vi "XNET Fill In Error Info Ex.vi"(0 "error xnet":errorcluster, 11 "error in":errorcluster) -> (15 "error out":errorcluster)   [LabVIEW 2018]
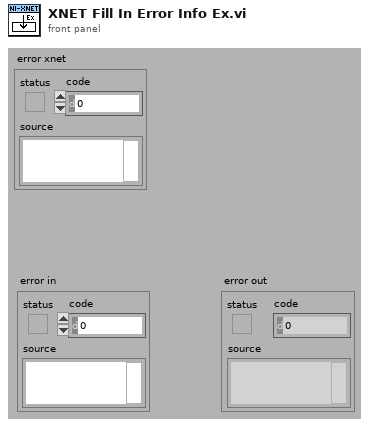
[diagram p1: front panel]
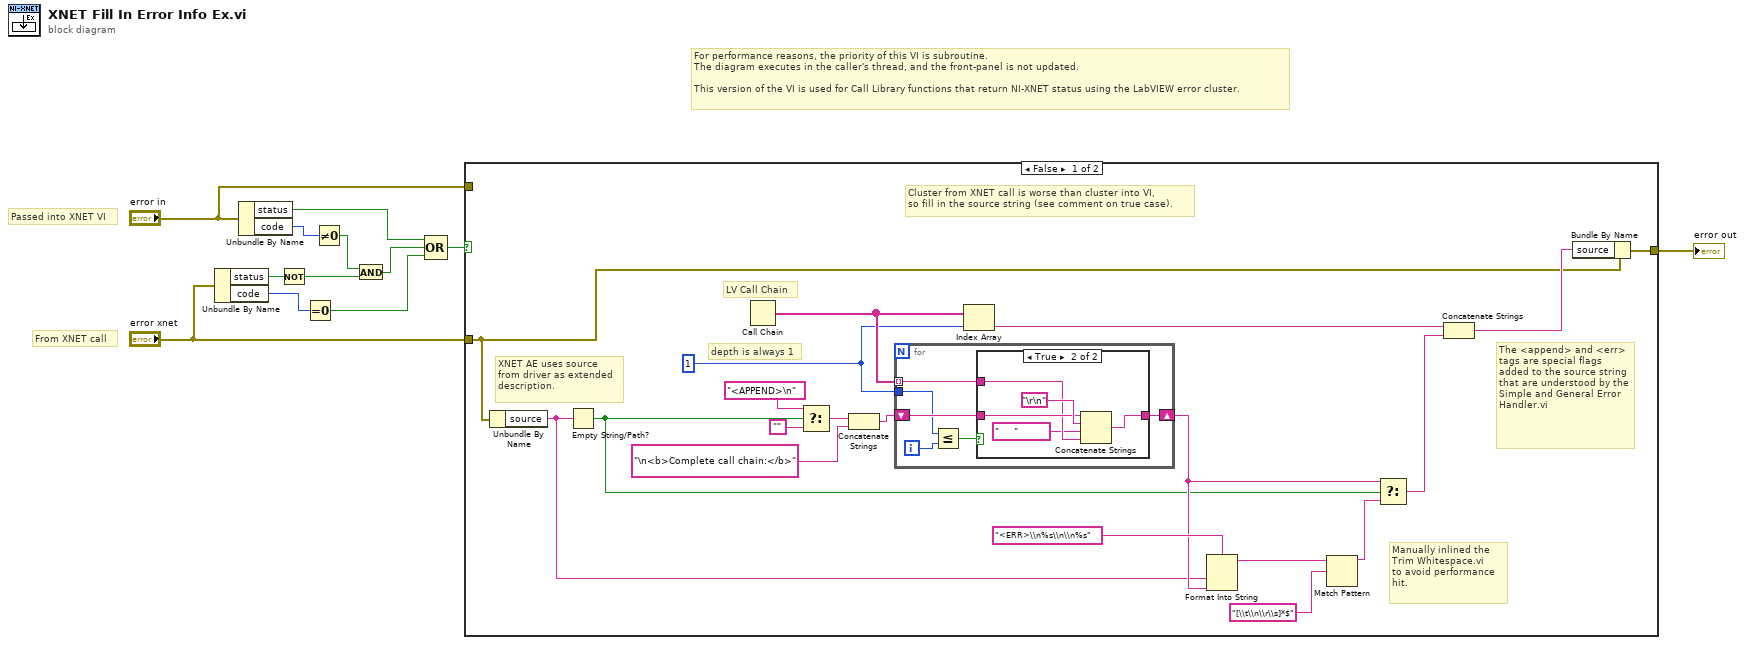
[diagram p0: block diagram]
diagram:
  # "From XNET call"
  # "Passed into XNET VI"
  # "For performance reasons, the priority of this VI is subroutine.\nThe diagram executes in the caller's thread, and the front-panel is not updated.\n\nThis version of the VI is used for Call Library functions that return NI-XNET status using the LabVIEW error cluster."
  n1 = Unbundle By Name("error xnet") -> ("status"=w4:bool, "code"=w2:i32)
  n2 = Unbundle By Name("error in") -> ("status"=w9:bool, "code"=w8:i32)
  n3 = Not(x=w4) -> (.not. x?=w3:bool)
  n4 = Equal To 0?(x=w2) -> (x = 0?=w1:bool)
  n5 = Not Equal To 0?(x=w8) -> (x != 0?=w5:bool)
  n6 = And(x=w5, y=w3) -> (x .and. y?=w6:bool)
  n7 = Compound Arithmetic op=OR(w9, w6, w1) -> (w10:bool)
  n8 = case shown="False" w10 {
    tunnel: [w31 w44] -> w12
    tunnel: "error in" -> [_ w44]
    tunnel: "error xnet" -> [w14 _]
    frame False {
      w15 = 1 ("depth (1)")
      # "LV Call Chain"
      # "XNET AE uses source\nfrom driver as extended\ndescription."
      # "Cluster from XNET call is worse than cluster into VI,\nso fill in the source string (see comment on true case)."
      # "depth is always 1"
      # "Manually inlined the\nTrim Whitespace.vi\nto avoid performance\nhit."
      # "The <append> and <err> tags are special flags added to the source string that are understood by the Simple and General Error Handler.vi"
      n9 = Unbundle By Name(w14) -> ("source"=w13:string)
      n10 = Empty String/Path?(string/path=w13) -> (empty?=w26:bool)
      n11 = Call Chain() -> (call chain=w16:string[])
      n12 = Select(t="<APPEND>\n", s=w26, f="") -> (s? t:f=w17:string)
      n13 = Concatenate Strings(w17, "\n<b>Complete call chain:</b>" ("call chain header")) -> (w20:string)
      n14 = for {
        tunnel: w16 -> [w35] mode=indexing
        shift-right: [w37] -> w28
        shift-left: w20 -> [w36]
        tunnel: w15 -> [w32]
        i -> [w33]
        n15 = Less Or Equal?(x=w32, y=w33) -> (x <= y?=w34:bool)
        n16 = case shown="True" w34 {
          tunnel: [w38 w43] -> w37
          tunnel: w36 -> [w38 w41]
          tunnel: w35 -> [_ w40]
          frame False {
          }
          frame True {
            n17 = Concatenate Strings(w41, "\r\n", "     ", w40) -> (w43:string)
          }
        }
      }
      n18 = Index Array(array=w16, index=w15) -> (element=w22:string)
      n19 = Format Into String(format string="<ERR>\\n%s\\n\\n%s", w13, w28) -> (resulting string=w24:string)  [unwired: 2 in, 1 out]
      n20 = Match Pattern(string=w24, regular expression="[\\t\\n\\r\\s]*$") -> (before substring=w23:string)  [unwired: 1 in, 3 out]
      n21 = Select(t=w28, s=w26, f=w23) -> (s? t:f=w27:string)
      n22 = Concatenate Strings(w22, w27) -> (w30:string)
      n23 = Bundle By Name(cluster=w14, "source"=w30) -> (w31:errorcluster)
    }
    frame True {
      # "Cluster from XNET call is not worse than cluster into VI,\nso do nothing.\n\nError is status==T.\nWarning is status==F code!=0.\nSuccess is status==F code==0.\n\nError is worse than Warning.\nWarning is worse than Success"
    }
  }
  "error out" <- w12
